vi "Get DLL Path.vi"() -> (2 "slscsl DLL Path":path)   [LabVIEW 2015, in "slscsl.lvclass"]
uses:
  slscsl.lvclass
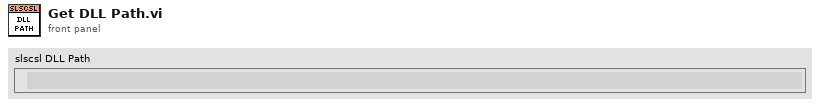
[diagram p1: front panel]
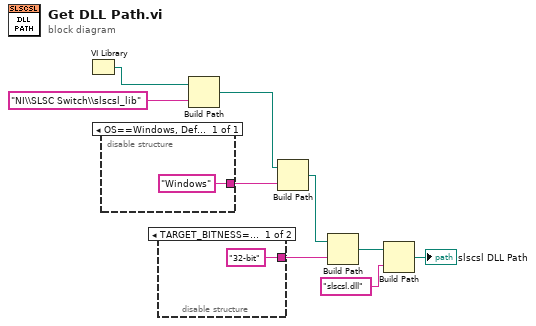
[diagram p0: block diagram]
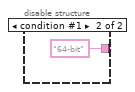
[diagram p2: hidden frame]
diagram:
  n1 = VI Library() -> (path=w1:path)
  n2 = disable-structure shown="OS==Windows, Default" {
    disable-tunnel: ["Windows" ("name or relative path")] -> w6
    frame condition #0 (active) {
    }
  }
  n3 = disable-structure shown="TARGET_BITNESS==32, Default" {
    disable-tunnel: ["32-bit" ("name or relative path") "64-bit" ("name or relative path")] -> w8
    frame condition #0 (active) {
    }
    frame condition #1 {
    }
  }
  n4 = Build Path(base path=w1, name or relative path="NI\\SLSC Switch\\slscsl_lib") -> (appended path=w7:path)
  n5 = Build Path(base path=w7, name or relative path=w6) -> (appended path=w5:path)
  n6 = Build Path(base path=w5, name or relative path=w8) -> (appended path=w4:path)
  n7 = Build Path(base path=w4, name or relative path="slscsl.dll") -> (appended path=→"slscsl DLL Path":path)
